vi "LUT_VITLogo.vi"() -> (0 "Init Data Out":fxp<+,12,12>[](array[numeric]))   [LabVIEW 2018]
panel:
  out "1/4":i32
  out "number of columns":i32
  out "number of rows":i32
  out "Original":picture
  out "Quotient":i32
  out "Remainder (Must be 0)":i32
  out "TotalPixels":i32
  out "Init Data Out size":i32
  # "For Initialization VI requirements and help, please read directions located on Block Diagram."
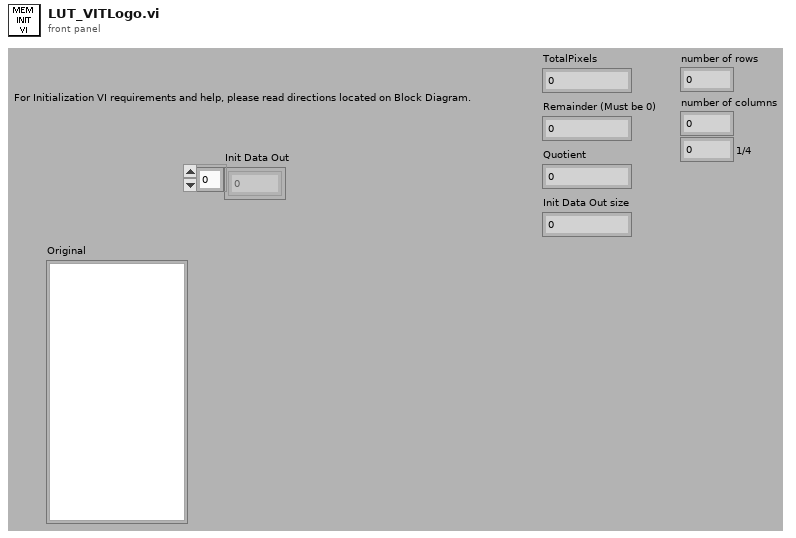
[diagram p1: front panel]
types:
  T1 = typedef "imagedata.ctl" = cluster{"image type":i32, "image depth":i32, "image":u8[], "mask":u8[], "colors":u32[], "Rectangle":cluster{"left":i16, "top":i16, "right":i16, "bottom":i16}}
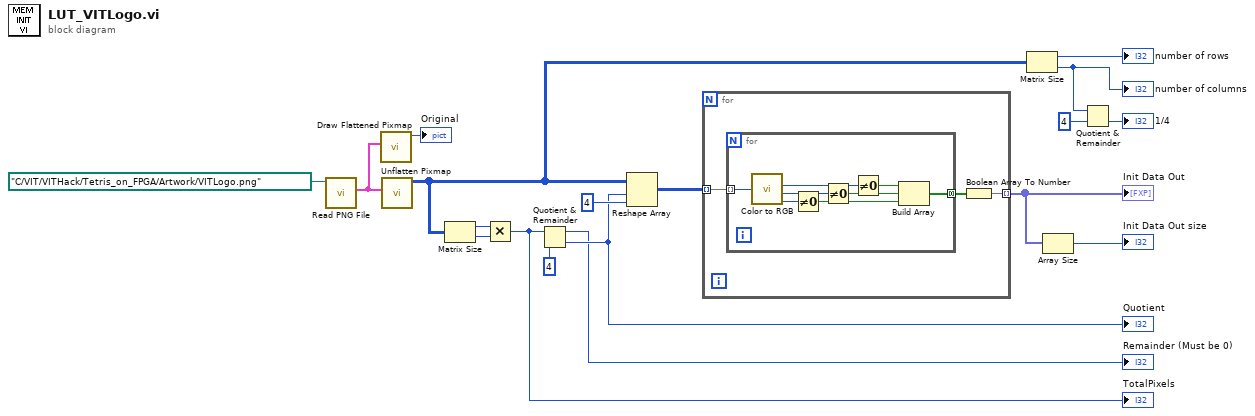
[diagram p0: block diagram]
diagram:
  n1 = call <vilib>:"Read PNG File.vi"("path to PNG file"=path "C:/VIT/VITHack/Tetris_on_FPGA/Artwork/VITLogo.png") -> ("image data"=w8:T1)  [unwired: 8 in, 2 out]
  n2 = call <vilib>:"Draw Flattened Pixmap.vi"("image data"=w8) -> ("new picture"=→"Original":picture)  [unwired: 8 in]
  n3 = call <vilib>:"Unflatten Pixmap.vi"("image data"=w8) -> ("24-bit pixmap"=w4:u32[][])  [unwired: 4 in, 6 out]
  n4 = Matrix Size(0:w4) -> (1:w11:i32, 2:w10:i32)
  n5 = Multiply(x=w11, y=w10) -> (x*y=w16:i32)
  "TotalPixels" <- w16
  n6 = Quotient & Remainder(x=w16, y=4) -> (x-y*floor(x/y)=→"Remainder (Must be 0)":i32, floor(x/y)=w14:i32)
  "Quotient" <- w14
  n7 = Reshape Array(w4, w14, 4 ("dimension size")) -> (w6:u32[][])
  n8 = for {
    tunnel: w6 -> [w21] mode=indexing
    tunnel: [w20] -> w9 mode=indexing
    n9 = for {
      tunnel: w21 -> [w29] mode=indexing
      tunnel: [w22] -> w19 mode=concatenating
      n10 = call <vilib>:"Color to RGB.vi"("Color"=w29) -> ("R"=w26:u8, "G"=w27:u8, "B"=w28:u8)  [unwired: 1 out]
      n11 = Not Equal To 0?(x=w28) -> (x != 0?=w23:bool)
      n12 = Not Equal To 0?(x=w27) -> (x != 0?=w24:bool)
      n13 = Not Equal To 0?(x=w26) -> (x != 0?=w25:bool)
      n14 = Build Array(w25, w24, w23) -> (w22:bool[])
    }
    n15 = Boolean Array To Number(Boolean array=w19) -> (number=w20:fxp<+,12,12>)
  }
  "Init Data Out" <- w9
  n16 = Matrix Size(0:w4) -> (1:→"number of rows":i32, 2:w3:i32)
  "number of columns" <- w3
  n17 = Array Size(array=w9) -> (size(s)=→"Init Data Out size":i32)
  n18 = Quotient & Remainder(x=w3, y=4) -> (floor(x/y)=→"1/4":i32)  [unwired: 1 out]
